vi "XML File.vi"(8 "error in (no error)":errorcluster, 9 "Action":T1) -> (0 "error out":errorcluster, 1 "Output":string)   [LabVIEW 2014, in "CD model script.lvlib"]
doc: "Constants, which are necessary for the custom device <B>XML file</B>."
uses:
  CD model script.lvlib
  Constants TypDef/XML File.ctl
  Constants TypDef/Common.ctl
  Common.vi
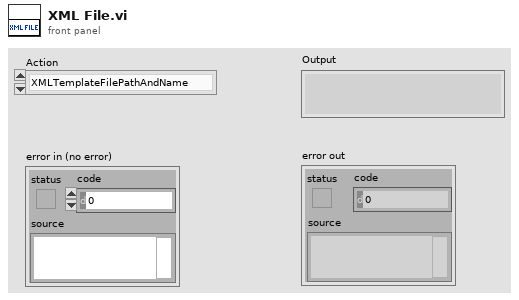
[diagram p1: front panel]
types:
  T1 = typedef "CD model script.lvlib/XML File.ctl" = enum16{"XMLTemplateFilePathAndName", "XMLTimingAndSyncFileName", "XMLCustomDeviceFileName"}
  T2 = typedef "CD model script.lvlib/Common.ctl" = enum16{"ProjectName", "TemplatesFolderName", "ProjectTemplatePathAndName", "ReadmeTemplatePathAndName", "TimingAndSyncFolderName", "CustomDeviceFolderName"}
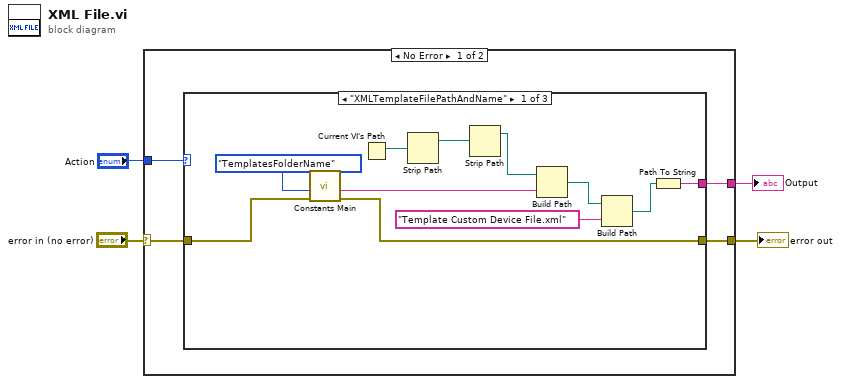
[diagram p0: block diagram]
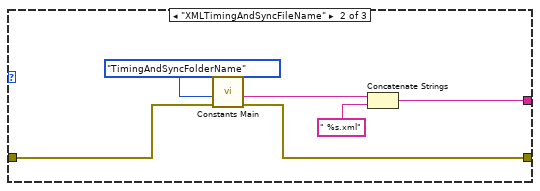
[diagram p2: hidden frame]
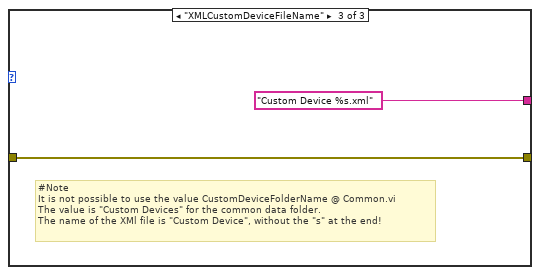
[diagram p3: hidden frame]
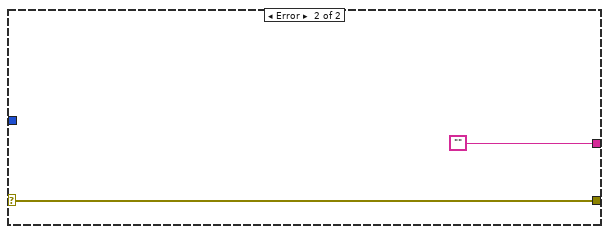
[diagram p4: hidden frame]
diagram:
  n1 = case shown="No Error" "error in (no error)" {
    selector: "error in (no error)" -> [w6 w29]
    tunnel: [w5 w29] -> w3
    tunnel: [w7 ""] -> w2
    tunnel: "Action" -> [w8 _]
    frame No Error {
      n2 = case shown="\"XMLTemplateFilePathAndName\"" w8 {
        tunnel: [w17 w20 "Custom Device %s.xml" ("format string")] -> w7
        tunnel: w6 -> [w16 w24 w27]
        tunnel: [w15 w21 w27] -> w5
        frame "XMLTemplateFilePathAndName" {
          n3 = call-poly "Constants Main.vi"("error in (no error)"=w16, "Action"=Common."TemplatesFolderName") -> ("error out"=w15:errorcluster, "Output"=w18:string)  [unwired: 8 in]
          n4 = Current VI's Path() -> (path=w11:path)
          n5 = Strip Path(path=w11) -> (stripped path=w10:path)  [unwired: 1 out]
          n6 = Strip Path(path=w10) -> (stripped path=w9:path)  [unwired: 1 out]
          n7 = Build Path(base path=w9, name or relative path=w18) -> (appended path=w14:path)
          n8 = Build Path(base path=w14, name or relative path="Template Custom Device File.xml" ("format string")) -> (appended path=w12:path)
          n9 = Path To String(path=w12) -> (string=w17:string)
        }
        frame "XMLTimingAndSyncFileName" {
          n10 = call-poly "Constants Main.vi"("error in (no error)"=w24, "Action"=Common."TimingAndSyncFolderName") -> ("error out"=w21:errorcluster, "Output"=w23:string)  [unwired: 8 in]
          n11 = Concatenate Strings(w23, " %s.xml" ("format string")) -> (w20:string)
        }
        frame "XMLCustomDeviceFileName" {
          # "#Note\nIt is not possible to use the value CustomDeviceFolderName @ Common.vi\nThe value is \"Custom Devices\" for the common data folder.\nThe name of the XMl file is \"Custom Device\", without the \"s\" at the end!"
        }
      }
    }
    frame Error {
    }
  }
  "error out" <- w3
  "Output" <- w2
